vi "Get Sender.vi"(11 "Last Ack Msg in":refnum<class "Last Ack Msg.lvclass">) -> (2 "Sender":refnum<class "Sender.lvclass">)   [LabVIEW 2020, in "jettl.lvlib" / "Last Ack Msg.lvlib" / "Last Ack Msg.lvclass"]
uses:
  Last Ack Msg.lvclass
  Sender/Sender/Sender.lvclass
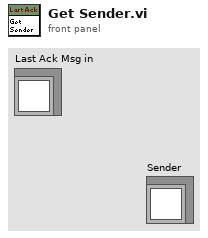
[diagram p1: front panel]
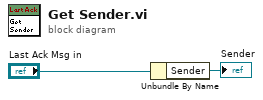
[diagram p0: block diagram]
diagram:
  n1 = Unbundle By Name("Last Ack Msg in") -> ("Sender"=→"Sender":refnum<class "Sender.lvclass">)
